vi "SE_HV200.constructor.vi"(0 "name":string, 2 "data in":string, 5 "error in(no error)":errorcluster) -> (14 "i ref out":refnum<vi>, 16 "data out":string, 19 "error out":errorcluster)   [LabVIEW 2014, in "SE_HV200.lvlib"]
doc: "High Voltage power supply FUG-HCN. This power supply can deliver upto 65KV. This class uses an instrument driver that is available via http://labview.gsi.de/driver.htm. The device is connected via GPIB. Finally, this device talks to a GPIB driver that must be installed on your system. Whenever a new frequency or amplitude value is set, that value is sent to the DSCInterface process for trending.\n\nauthors: Frank Herfurth (CERN) and Sumit Saxena\nadapted to CS v3 by: R.Savreux, CERN\n\nLicense Agreement for this software:\n\nCopyright (C)\nGesellschaft für Schwerionenforschung, GSI\nPlanckstr. 1\n64291 Darmstadt\nGermany\n\nContact: D.Beck@gsi.de \n\nThis program is free software; you can redistribute it and/or modify it under the terms of the \nGNU General Public License as published by the Free Software Foundation; either version 2 of \nthe license, or (at your option) any later version.\n\nThis program is distributed in the hope that it will be useful, but WITHOUT ANY WARRANTY; \nwithout even the implied warranty of MERCHANTABILITY or FITNESS FOR A PARTICULAR PURPOSE. See the GNU General License for more details (http://www.gnu.org).\n\nGesellschaft für Schwerionenforschung, GSI\nPlanckstr. 1, 64291 Darmstadt, Germany\nFor all questions and ideas contact: M.Richter@gsi.de, H.Brand@gsi.de or D.Beck@gsi.de.\nLast update: 16-JUN-2004"
uses:
  SE_HV200.lvlib
  CSCore/BaseProcess/BaseProcess.lvlib
  CSCore/CSSystem/CSSystemLib/CSSystemLib.lvlib
  CSlibraries-extern/DimLVEvent/LVDimInterface/LVDimInterface.lvlib
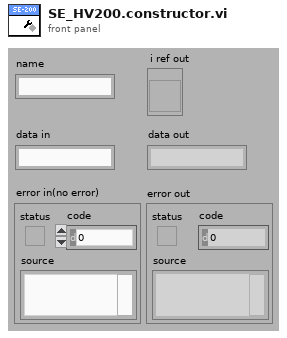
[diagram p1: front panel]
types:
  T1 = enum16{"SetAttribute", "GetAttribute", "CreateAttribute", "DestroyAttribute", "DestroyAllAtributes"}
  T2 = typedef "BaseProcess.lvlib/BaseProcess.i attribute.ctl" = cluster{"EventStatus":string, "EventError":i32, "PresetEvtWatchD":i32, "PresetPdcWatchD":i32, "EventTimeout":i32, "PeriodicInterval":i32, "Interface":string[], "Address":string[], "Special":string[], "PeriodicError":i32, "PeriodicStatus":string, "SuperProc":string, "Descriptors":T3[], "CaseRef":refnum<vi>, "PdcRef":refnum<vi>, "Thread Ref":refnum<vi>, "eventErrorID":i32, "eventStatusID":i32, "periodicErrorID":i32, "periodicStatusID":i32, "pdcCtrID":i32}
  T3 = typedef "BaseProcess.lvlib/BaseProcess.descriptor definition.ctl" = cluster{"selector":string, "descriptor":T4}
  T4 = typedef "BaseProcess.lvlib/BaseProcess.descriptor string definition.ctl" = string
  T5 = typedef "SE_HV200.lvlib/SE_HV200.i attribute.ctl" = cluster{"SetStatus":bool, "actVoltageID":i32, "VISA resource name in":refnum<visa-resource-name>, "Device name":string, "PSRange":i32, "nomVoltageID":i32, "actStatusID":i32, "NomVoltage":dbl[], "ActVoltage":dbl[], "DefaultChannel":i32}
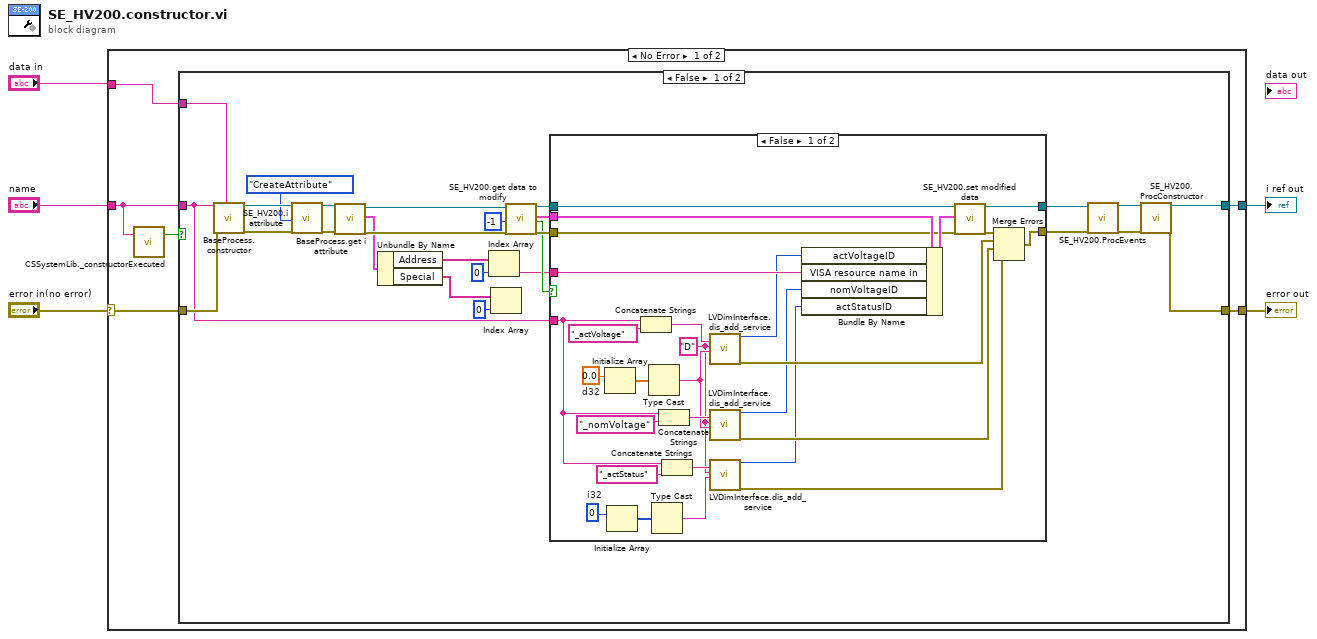
[diagram p0: block diagram]
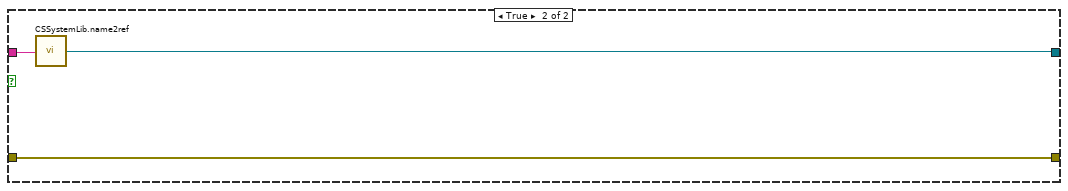
[diagram p3: hidden frame]
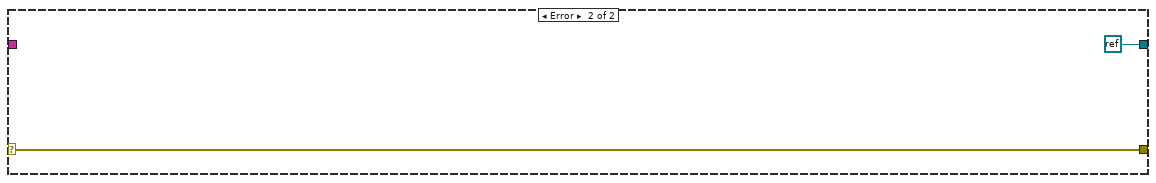
[diagram p4: hidden frame]
diagram:
  n1 = case shown="No Error" "error in(no error)" {
    selector: "error in(no error)" -> [w9 w73]
    tunnel: "name" -> [w8 _]
    tunnel: [w11 refnum<k0> refnum ("i ref out")] -> w4
    tunnel: [w10 w73] -> w3
    tunnel: "data in" -> [w6 _]
    frame No Error {
      n2 = call "CSSystemLib._constructorExecuted.vi"("name"=w8) -> ("constructor executed?"=w7:bool)  [unwired: 18 in]
      n3 = case shown="False" w7 {
        tunnel: [w34 w70] -> w11
        tunnel: [w33 w69] -> w10
        tunnel: w9 -> [w32 w69]
        tunnel: w8 -> [w24 w71]
        tunnel: w6 -> [w23 _]
        frame False {
          n4 = call "BaseProcess.constructor.vi"("name"=w24, "data in"=w23, "error in (no error)"=w32) -> ("i ref out"=w38:refnum<vi>, "error out"=w22:errorcluster)  [unwired: 14 in, 1 out]
          n5 = call "SE_HV200.i attribute.vi"("VI Refnum"=w38, "Action"=T1."CreateAttribute", "error in (no error)"=w22) -> ("VI Refnum out"=w19:refnum<vi>, "error out"=w18:errorcluster)  [unwired: 14 in, 1 out]
          n6 = call "BaseProcess.get i attribute.vi"("i ref in"=w19, "error in (no error)"=w18) -> ("i ref out"=w16:refnum<vi>, "i attribute"=w15:T2, "error out"=w17:errorcluster)  [unwired: 15 in]
          n7 = Unbundle By Name(w15) -> ("Address"=w14:string[], "Special"=w12:string[])
          n8 = Index Array(array=w14, index=0) -> (element=w20:string)
          n9 = Index Array(array=w12, index=0) -> ()  [unwired: 1 out]
          n10 = call "SE_HV200.get data to modify.vi"("i ref in"=w16, "ms timeout (10000)"=-1, "error in (no error)"=w17) -> ("i ref out"=w29:refnum<vi>, "i attribute"=w30:T5, "timed out"=w25:bool, "error out"=w28:errorcluster)  [unwired: 13 in]
          n11 = case shown="False" w25 {
            tunnel: w30 -> [w66 _]
            tunnel: w29 -> [w65 w68]
            tunnel: w28 -> [w63 w67]
            tunnel: [w62 w68] -> w27
            tunnel: [w60 w67] -> w26
            tunnel: w24 -> [w49 _]
            tunnel: w20 -> [w56 _]
            frame False {
              w44 = 0  # i32
              w55 = 0.0  # d32
              w46 = "D" ("typeDescriptor")
              n12 = Initialize Array(w55) -> (w54:dbl[])  [unwired: 1 in]
              n13 = Initialize Array(w44) -> (w43:i32[])  [unwired: 1 in]
              n14 = Concatenate Strings(w49, "_actVoltage" ("string")) -> (w59:string)
              n15 = Type Cast(x=w54) -> (*(type *) &x=w47:string)  [unwired: 1 in]
              n16 = Type Cast(x=w43) -> (*(type *) &x=w42:string)  [unwired: 1 in]
              n17 = Concatenate Strings(w49, "_nomVoltage" ("string")) -> (w52:string)
              n18 = Concatenate Strings(w49, "_actStatus" ("string")) -> (w48:string)
              n19 = call "LVDimInterface.dis_add_service.vi"("serviceName"=w59, "typeDescriptor"=w46, "data"=w47) -> ("my_serviceID"=w41:i32, "error out"=w57:errorcluster)  [unwired: 15 in]
              n20 = call "LVDimInterface.dis_add_service.vi"("serviceName"=w52, "typeDescriptor"=w46, "data"=w47) -> ("my_serviceID"=w40:i32, "error out"=w51:errorcluster)  [unwired: 15 in]
              n21 = call "LVDimInterface.dis_add_service.vi"("serviceName"=w48, "typeDescriptor"=w46, "data"=w42) -> ("my_serviceID"=w39:i32, "error out"=w45:errorcluster)  [unwired: 15 in]
              n22 = Bundle By Name(cluster=w66, "actVoltageID"=w41, "VISA resource name in"=w56, "nomVoltageID"=w40, "actStatusID"=w39) -> (w64:T5)
              n23 = call "SE_HV200.set modified data.vi"("i ref in"=w65, "i attribute"=w64, "error in (no error)"=w63) -> ("i ref out"=w62:refnum<vi>, "error out"=w61:errorcluster)  [unwired: 15 in]
              n24 = Merge Errors(w61, w57, w51, w45) -> (w60:errorcluster)
            }
            frame True {
            }
          }
          n25 = call "SE_HV200.ProcEvents.vi"("i ref in"=w27, "error in"=w26) -> ("i ref out"=w36:refnum<vi>, "error out"=w35:errorcluster)  [unwired: 16 in]
          n26 = call "SE_HV200.ProcConstructor.vi"("i ref in"=w36, "error in (no error)"=w35) -> ("i ref out"=w34:refnum<vi>, "error out"=w33:errorcluster)  [unwired: 16 in]
        }
        frame True {
          n27 = call "CSSystemLib.name2ref.vi"("name"=w71) -> ("obj refnum"=w70:refnum<vi>)
        }
      }
    }
    frame Error {
    }
  }
  "i ref out" <- w4
  "error out" <- w3
